vi "Write Pressure.vi"(8 "error in (no error)":errorcluster, 10 "Pressure":cluster{"Start":dbl, "Final":dbl}, 11 "P Cal Builder in":refnum<class "P Cal Builder.lvclass">) -> (0 "error out":errorcluster, 3 "P Cal Builder out":refnum<class "P Cal Builder.lvclass">)   [LabVIEW 2015, in "P Cal Builder.lvclass"]
uses:
  P Cal Builder.lvclass
  P Cal Builder.lvclass/P Cal Builder.ctl
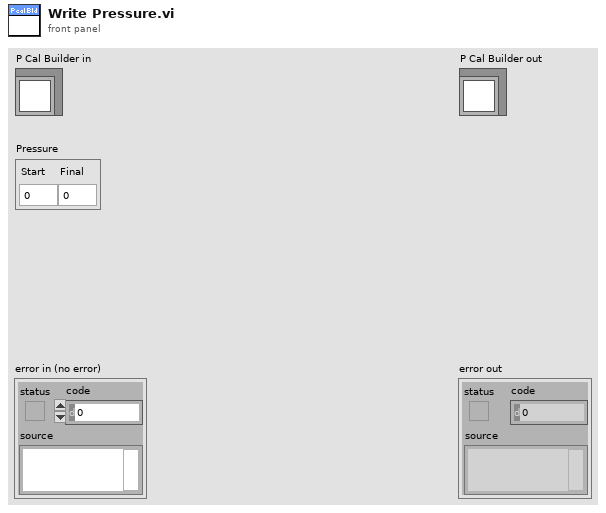
[diagram p1: front panel]
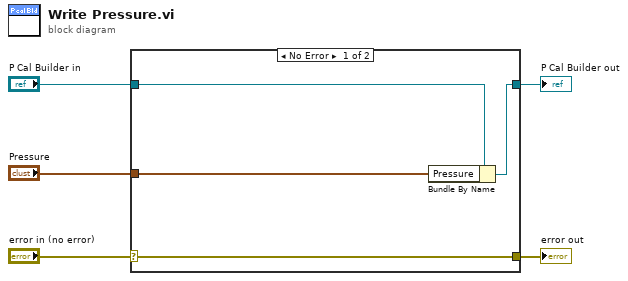
[diagram p0: block diagram]
diagram:
  n1 = case shown="No Error" "error in (no error)" {
    selector: "error in (no error)" -> [w9 w10]
    tunnel: [w9 w10] -> w4
    tunnel: [w7 w11] -> w2
    tunnel: "P Cal Builder in" -> [w8 w11]
    tunnel: "Pressure" -> [w6 _]
    frame No Error {
      n2 = Bundle By Name(cluster=w8, "Pressure"=w6) -> (w7:refnum<class "P Cal Builder.lvclass">)
    }
    frame Error {
    }
  }
  "error out" <- w4
  "P Cal Builder out" <- w2
